vi "Word - Save And SaveAs Docuement Tests.vi"(8 "error in (no error)":errorcluster) -> (0 "error out":errorcluster)   [LabVIEW 2017]
uses:
  src/LabVIEW NPOI/MS-Word/MS-Word.lvclass
  C:/Users/Neo/Desktop/Dev_Tools_BR/LabVIEW_NPOI/src/LabVIEW NPOI/Document/Document.lvclass
  src/LabVIEW NPOI/Document/Document.lvclass/Document.ctl
  src/LabVIEW NPOI/Document/Get FilePath.vi
  src/LabVIEW NPOI/Document/Get Word Document Reference.vi
  <vilib>/addons/_JKI Toolkits/Caraya/classes/Assert/Assert Not Error.vi
  <vilib>/addons/_JKI Toolkits/Caraya/classes/Assert/Assert False.vi
  <vilib>/addons/_JKI Toolkits/Caraya/classes/Assert/Assert True.vi
  C:/Users/Neo/Desktop/Dev_Tools_BR/LabVIEW_NPOI/src/lib/NPOI 2.1.1/NPOI.OOXML.dll
  src/lib/NPOI 2.1.1/NPOI.OOXML.dll
  src/LabVIEW NPOI/Document/Document.lvclass
  <vilib>/addons/_JKI Toolkits/Caraya/classes/Test/Test.lvclass
  <vilib>/addons/_JKI Toolkits/Caraya/classes/Assert/Assert.lvclass
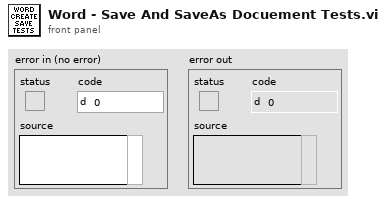
[diagram p1: front panel]
types:
  T1 = enum16{"open", "replace", "create", "open or create", "replace or create", "replace or create with confirmation"}
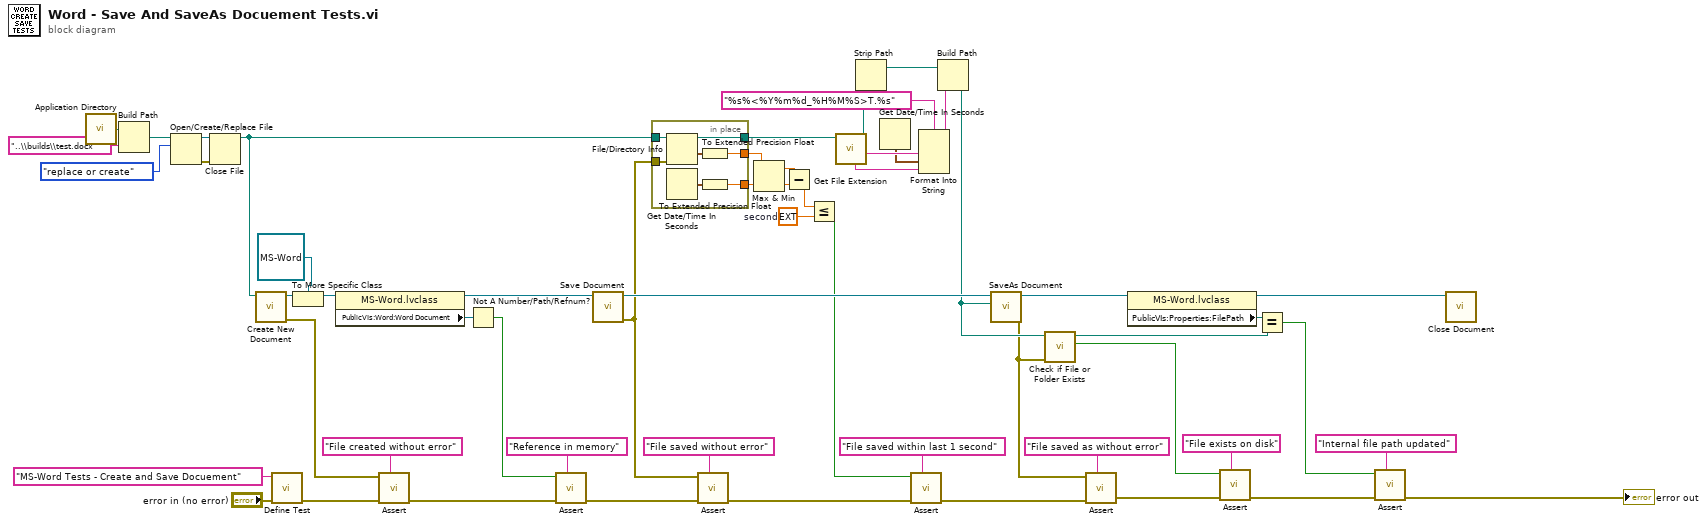
[diagram p0: block diagram]
diagram:
  w5 = ext 1.0  # second
  n1 = call <vilib>:"Application Directory.vi"() -> ("Application Directory"=w29:path)
  n2 = Build Path(base path=w29, name or relative path="..\\builds\\test.docx" ("string")) -> (appended path=w27:path)
  n3 = Open/Create/Replace File(file path (use dialog)=w27, operation (0:open)=T1."replace or create") -> (refnum out=w40:refnum<file>, error out=w41:errorcluster)  [unwired: 4 in, 1 out]
  n4 = Close File(refnum=w40, error in=w41) -> (path=w3:path)  [unwired: 1 out]
  n5 = call "Create New Document.vi"("File Path"=w3) -> ("error out"=w53:errorcluster, "Document out"=w56:refnum<class "Document.lvclass">)  [unwired: 9 in]
  n6 = call <vilib>:"Define Test.vi"("error in (no error)"="error in (no error)", "Label (VI Title)"="MS-Word Tests - Create and Save Docuement") -> ("error out"=w55:errorcluster)  [unwired: 9 in]
  n7 = To More Specific Class(target class=refnum<class "MS-Word.lvclass"> refnum ("LabVIEW NPOI.lvlib:MS-Word.lvclass"), reference=w56) -> (specific class reference=w2:refnum<class "MS-Word.lvclass">)  [unwired: 1 in, 1 out]
  n8 = property class="MS-Word.lvclass"(reference=w2) -> (reference out=w47:refnum<class "MS-Word.lvclass">, "PublicVIs:Word:Word Document"=w42:refnum<k24>)  [unwired: 1 in, 1 out]
  n9 = call-poly <vilib>:"Assert.vi"("Label"="File created without error", "error in (no error)"=w55, "Not Error?"=w53) -> ("error out"=w51:errorcluster)  [unwired: 8 in]
  n10 = Not A Number/Path/Refnum?(number/path/refnum=w42) -> (NaN/Path/Refnum?=w52:bool)
  n11 = call-poly <vilib>:"Assert.vi"("Label"="Reference in memory", "error in (no error)"=w51, "False?"=w52) -> ("error out"=w44:errorcluster)  [unwired: 8 in]
  n12 = call "Save Document.vi"("Document in"=w47) -> ("error out"=w38:errorcluster, "Document out"=w46:refnum<class "MS-Word.lvclass">)  [unwired: 9 in]
  n13 = in-place {
    in-place-border: w38 -> [w63]
    in-place-border: w3 -> [w62]
    in-place-border: [w61] -> w36
    in-place-border: [w58] -> w9
    in-place-border: [w57] -> w8
    n14 = File/Directory Info(path=w62, error in=w63) -> (path out=w61:path, last mod=w60:timestamp)  [unwired: 5 out]
    n15 = Get Date/Time In Seconds() -> (seconds since 1Jan1904=w59:timestamp)
    n16 = To Extended Precision Float(1:w60) -> (0:w58:ext)
    n17 = To Extended Precision Float(1:w59) -> (0:w57:ext)
  }
  n18 = call-poly <vilib>:"Assert.vi"("Label"="File saved without error", "error in (no error)"=w44, "Not Error?"=w38) -> ("error out"=w13:errorcluster)  [unwired: 8 in]
  n19 = Max & Min(x=w9, y=w8) -> (max(x,y)=w11:ext, min(x,y)=w10:ext)
  n20 = Subtract(x=w11, y=w10) -> (x-y=w7:ext)
  n21 = Less Or Equal?(x=w7, y=w5) -> (x <= y?=w6:bool)
  n22 = call <vilib>:"Get File Extension.vi"("file"=w36) -> ("filename without extension"=w35:string, "dup file"=w32:path, "unmodified file extension"=w33:string)  [unwired: 6 in, 2 out]
  n23 = Strip Path(path=w32) -> (stripped path=w31:path)  [unwired: 1 out]
  n24 = Get Date/Time In Seconds() -> (seconds since 1Jan1904=w26:timestamp)
  n25 = call-poly <vilib>:"Assert.vi"("Label"="File saved within last 1 second", "error in (no error)"=w13, "True?"=w6) -> ("error out"=w12:errorcluster)  [unwired: 8 in]
  n26 = Format Into String(format string="%s%<%Y%m%d_%H%M%S>T.%s", w35, w26, w33) -> (resulting string=w30:string)  [unwired: 2 in, 1 out]
  n27 = Build Path(base path=w31, name or relative path=w30) -> (appended path=w25:path)
  n28 = call "SaveAs Document.vi"("File Path"=w25, "Document in"=w46) -> ("error out"=w24:errorcluster, "Document out"=w37:refnum<class "MS-Word.lvclass">)  [unwired: 8 in]
  n29 = call <vilib>:"Check if File or Folder Exists.vi"("error in (no error)"=w24, "path"=w25) -> ("file or folder exists?"=w21:bool, "dup path"=w18:path)  [unwired: 7 in, 1 out]
  n30 = call-poly <vilib>:"Assert.vi"("Label"="File saved as without error", "error in (no error)"=w12, "Not Error?"=w24) -> ("error out"=w22:errorcluster)  [unwired: 8 in]
  n31 = property class="MS-Word.lvclass"(reference=w37) -> (reference out=w20:refnum<class "MS-Word.lvclass">, "PublicVIs:Properties:FilePath"=w19:path)  [unwired: 1 in, 1 out]
  n32 = call-poly <vilib>:"Assert.vi"("Label"="File exists on disk", "error in (no error)"=w22, "True?"=w21) -> ("error out"=w16:errorcluster)  [unwired: 8 in]
  n33 = Equal?(x=w19, y=w18) -> (x = y?=w14:bool)
  n34 = call-poly <vilib>:"Assert.vi"("Label"="Internal file path updated", "error in (no error)"=w16, "True?"=w14) -> ("error out"=→"error out":errorcluster)  [unwired: 8 in]
  n35 = call "Close Document.vi"("Document in"=w20) -> ()  [unwired: 10 in, 1 out]
